vi "MyFourth.vi"(8 "error in (no error)":errorcluster, 10 "path to JPEG file":path, 11 "Border":T1={"BG Blue Rmin"=0.0, "BG Blue Rmax "=24.0, " BG Blue Gmin"=0.0, "BG Blue Gmax"=49.0, "BG Blue Bmin "=100.0, "Bg Blue Bmax"=119.0}) -> (0 "error out":errorcluster, 3 "Bornes":cluster{i32, i32, "Ymin":i32, "Ymax":i32})   [LabVIEW 2025]
panel:
  out "Ymax":i32
  out "Ymin":i16
  out "Xmax":i32
  out "Xmin":i16
  out "coerced(x) 3":u8
  out "coerced(x) 2":u8
  out "coerced(x)":u8
  out "largeur = maxX of whole picture":i16
  out "hauter = maxY of whole picture":i16
  out "B":u8
  out "G":u8
  out "R":u8
  out "X crt":i32
  out "Y crt":i32
  out "24-bit pixmap":u32[][](array[numeric]) format="%x"
  # "Xmin"
  # "Xmax"
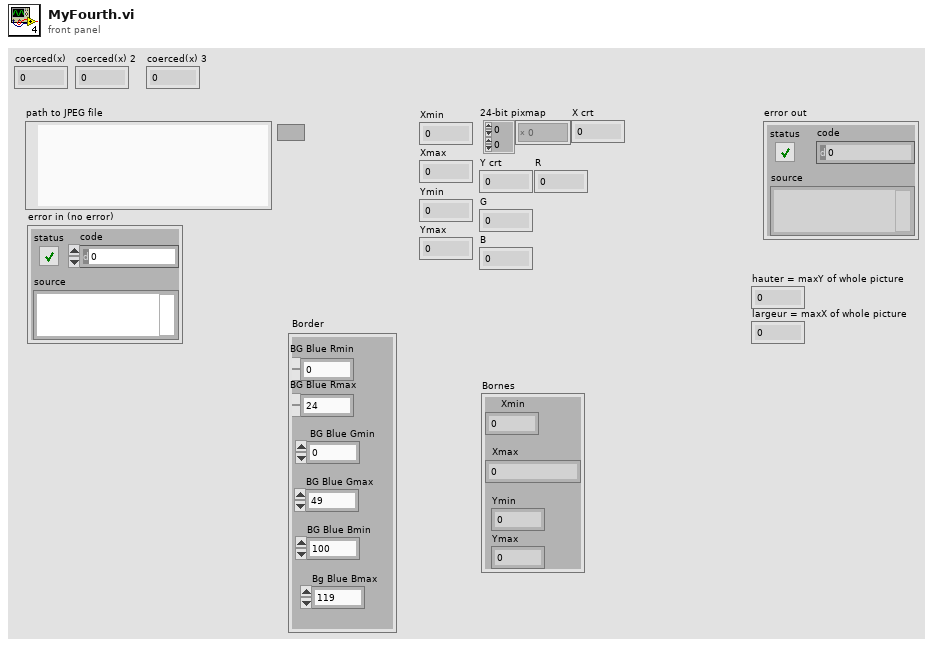
[diagram p1: front panel]
types:
  T1 = cluster{"BG Blue Rmin":dbl, "BG Blue Rmax ":dbl, " BG Blue Gmin":dbl, "BG Blue Gmax":dbl, "BG Blue Bmin ":dbl, "Bg Blue Bmax":dbl}
  T2 = typedef "imagedata.ctl" = cluster{"image type":i32, "image depth":i32, "image":u8[], "mask":u8[], "colors":u32[], "Rectangle":cluster{"left":i16, "top":i16, "right":i16, "bottom":i16}}
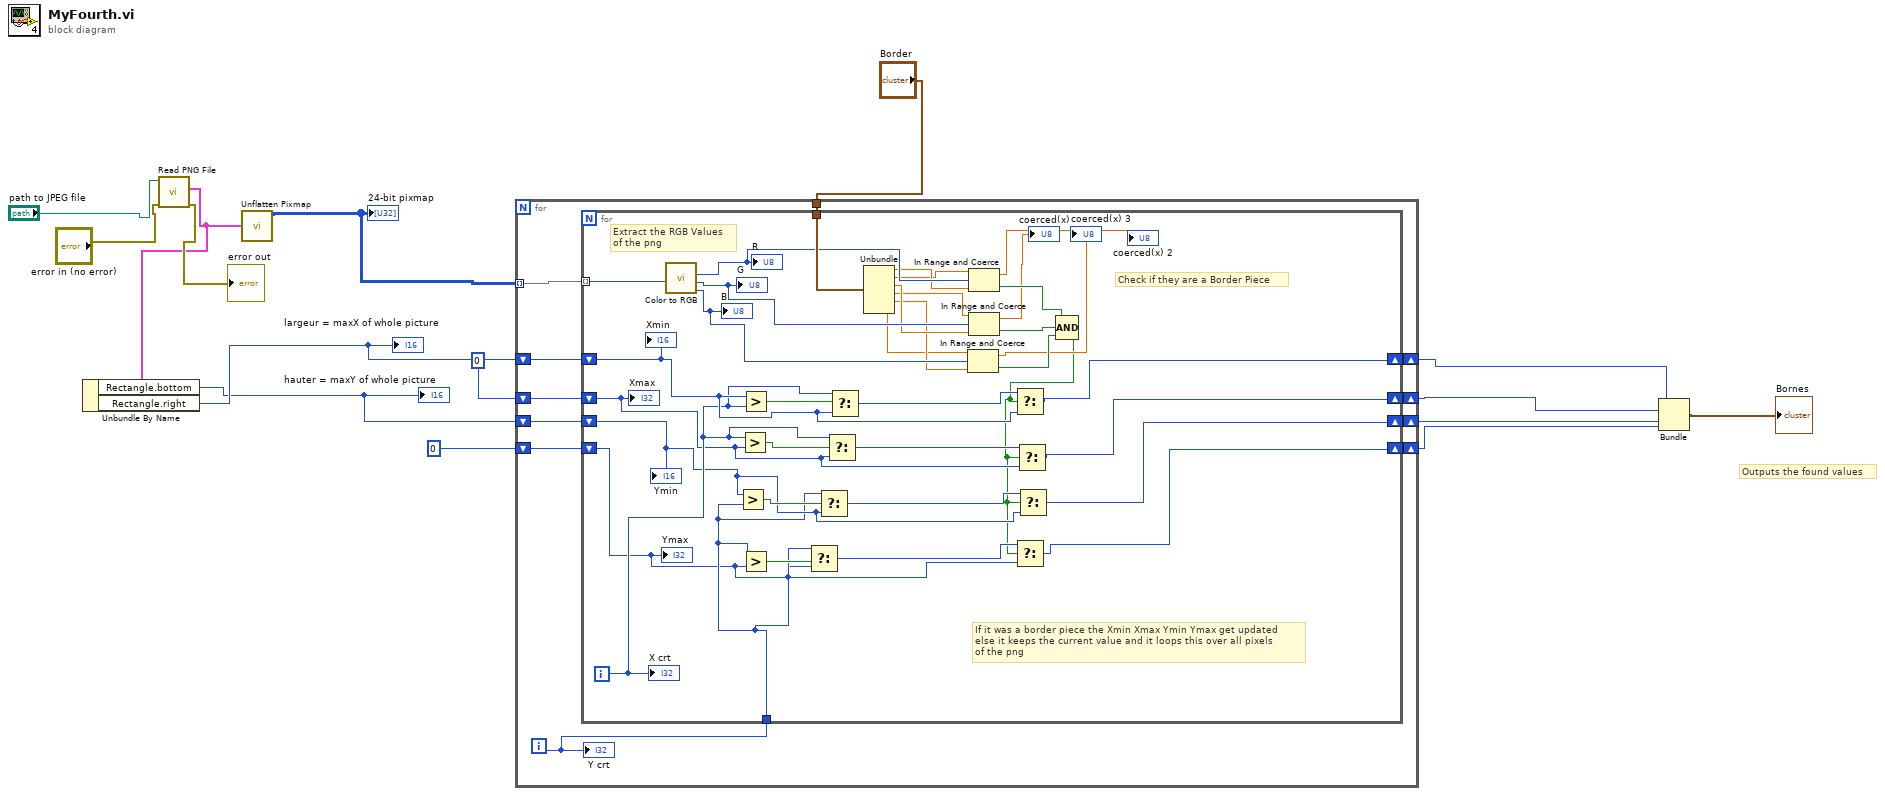
[diagram p0: block diagram]
diagram:
  # "Outputs the found values"
  n1 = call <vilib>:"Read PNG File.vi"("error in (no error)"="error in (no error)", "path to PNG file"="path to JPEG file") -> ("error out"=→"error out":errorcluster, "image data"=w9:T2)  [unwired: 7 in, 1 out]
  n2 = Unbundle By Name(w9) -> ("Rectangle.bottom"=w6:i16, "Rectangle.right"=w8:i16)
  "hauter = maxY of whole picture" <- w6
  "largeur = maxX of whole picture" <- w8
  n3 = call <vilib>:"Unflatten Pixmap.vi"("image data"=w9) -> ("24-bit pixmap"=w15:u32[][])  [unwired: 4 in, 6 out]
  "24-bit pixmap" <- w15
  n4 = for {
    tunnel: w15 -> [w26] mode=indexing
    tunnel: "Border" -> [w24]
    shift-right: [w19] -> w3
    shift-left: 0 -> [w22]
    shift-right: [w18] -> w1
    shift-left: 0 -> [w20]
    shift-right: [w17] -> w2
    shift-left: w6 -> [w21]
    shift-right: [w16] -> w4
    shift-left: w8 -> [w23]
    i -> [w25]
    n5 = for {
      tunnel: w26 -> [w62] mode=indexing
      tunnel: w25 -> [w31]
      tunnel: w24 -> [w61]
      shift-right: [w37] -> w19
      shift-left: w22 -> [w39]
      shift-right: [w33] -> w17
      shift-left: w21 -> [w34]
      shift-right: [w28] -> w18
      shift-left: w20 -> [w29]
      shift-right: [w38] -> w16
      shift-left: w23 -> [w43]
      i -> [w41]
      # "If it was a border piece the Xmin Xmax Ymin Ymax get updated\nelse it keeps the current value and it loops this over all pixels \nof the png"
      # "Check if they are a Border Piece"
      # "Extract the RGB Values\nof the png"
      n6 = call <vilib>:"Color to RGB.vi"("Color"=w62) -> ("R"=w60:u8, "G"=w59:u8, "B"=w58:u8)  [unwired: 1 out]
      "R" <- w60
      "G" <- w59
      "B" <- w58
      n7 = Greater?(x=w34, y=w31) -> (0:w36:bool)
      n8 = Greater?(x=w41, y=w39) -> (0:w42:bool)
      n9 = Greater?(x=w43, y=w41) -> (0:w45:bool)
      n10 = Greater?(x=w31, y=w29) -> (0:w32:bool)
      n11 = Select(t=w31, s=w32, f=w29) -> (s? t:f=w30:i32)
      n12 = Select(t=w31, s=w36, f=w34) -> (s? t:f=w35:i32)
      n13 = Select(t=w41, s=w42, f=w39) -> (s? t:f=w40:i32)
      n14 = Select(t=w41, s=w45, f=w43) -> (s? t:f=w44:i32)
      n15 = Unbundle(w61) -> ("BG Blue Rmin"=w51:dbl, "BG Blue Rmax"=w50:dbl, "BG Blue Gmin"=w49:dbl, "BG Blue Gmax"=w48:dbl, "BG Blue Bmin"=w47:dbl, "Bg Blue Bmax"=w46:dbl)
      n16 = In Range and Coerce(upper limit=w46, x=w58, lower limit=w47) -> (coerced(x)=→"coerced(x) 3":dbl, In Range?=w55:bool)
      n17 = In Range and Coerce(upper limit=w50, x=w60, lower limit=w51) -> (coerced(x)=→"coerced(x) 2":dbl, In Range?=w57:bool)
      n18 = In Range and Coerce(upper limit=w48, x=w59, lower limit=w49) -> (coerced(x)=→"coerced(x)":dbl, In Range?=w56:bool)
      n19 = Compound Arithmetic op=AND(w57, w56, w55) -> (w27:bool)
      n20 = Select(t=w44, s=w27, f=w43) -> (s? t:f=w38:i32)
      n21 = Select(t=w30, s=w27, f=w29) -> (s? t:f=w28:i32)
      n22 = Select(t=w40, s=w27, f=w39) -> (s? t:f=w37:i32)
      n23 = Select(t=w35, s=w27, f=w34) -> (s? t:f=w33:i32)
      "X crt" <- w41
      "Xmin" <- w43
      "Xmax" <- w39
      "Ymin" <- w34
      "Ymax" <- w29
    }
    "Y crt" <- w25
  }
  n24 = Bundle("right"=w4, w3, "bottom"=w2, w1) -> (→"Bornes":cluster{"right":i32, i32, "bottom":i32, i32})  [unwired: 1 in]
